vi "parseSpectralData.vi"(8 "error in (no error)":errorcluster, 11 "results-JSON string":string) -> (0 "error out":errorcluster, 2 "meta data":T1[][](array[typedef]), 3 "xyData":dbl[][][][](array[numeric]))   [LabVIEW 2023, in "CCD.lvclass"]
uses:
  CCD.lvclass
  CCDSpectralData.ctl
  81c9510d-da94-45eb-b341-4ac2c5dcdc17.vi
  <vilib>/JDP Science/JSONtext/Next JSON Value.vi
  <vilib>/JDP Science/JSONtext/String Subset.vi
  <vilib>/JDP Science/JSONtext/Parsing/Advance past next JSON Value (inlined COPY).vi
  <vilib>/JDP Science/JSONtext/Parsing/Advance past whitespace.vi
  <vilib>/JDP Science/JSONtext/Parsing/Advance past String.vi
  <vilib>/JDP Science/JSONtext/Parsing/Advance past Number.vi
  <vilib>/JDP Science/JSONtext/Parsing/Advance past Line Ending.vi
  <vilib>/JDP Science/JSONtext/Parsing/Parse Full Path or Item Name.vi
  <vilib>/JDP Science/JSONtext/Parsing/Advance past Array.vi
  <vilib>/JDP Science/JSONtext/Parsing/Advance past Object.vi
  <vilib>/JDP Science/JSONtext/support/Error Cluster From Code.vi
  <vilib>/JDP Science/JSONtext/Offset/Find Item Locations by Path.vi
  <vilib>/JDP Science/JSONtext/JSON text to Variant.vi
  <vilib>/JDP Science/JSONtext/LVClass Serializer/JSONtext LVClass Serializer.lvclass
  CCD.lvclass/CCD.ctl
  <vilib>/JDP Science/JSONtext/JSONtext.lvlib
panel:
  # "acquisition"
  # "ROI"
  # "x-pixel (wavelength)"
  # "unused"
  # "Connector Pane"
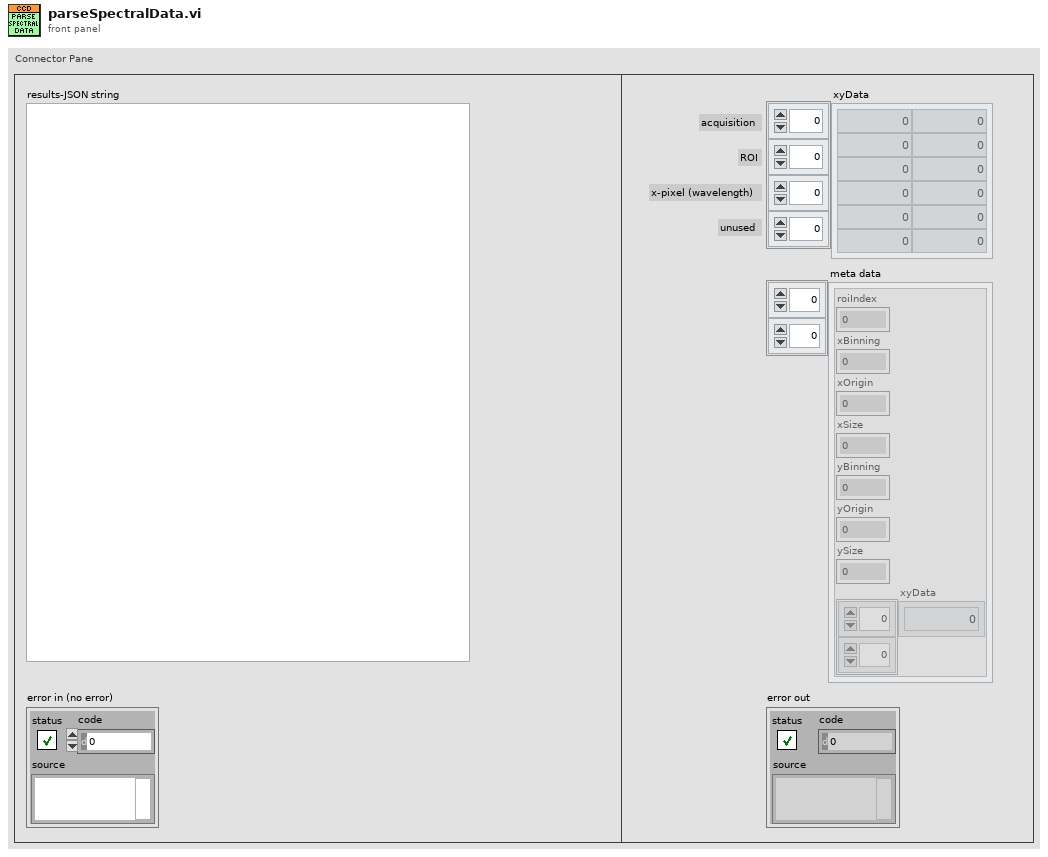
[diagram p1: front panel]
types:
  T1 = typedef "CCD.lvclass/CCDSpectralData.ctl" = cluster{"roiIndex":i32, "xBinning":i32, "xOrigin":i32, "xSize":i32, "yBinning":i32, "yOrigin":i32, "ySize":i32, "xyData":dbl[][]}
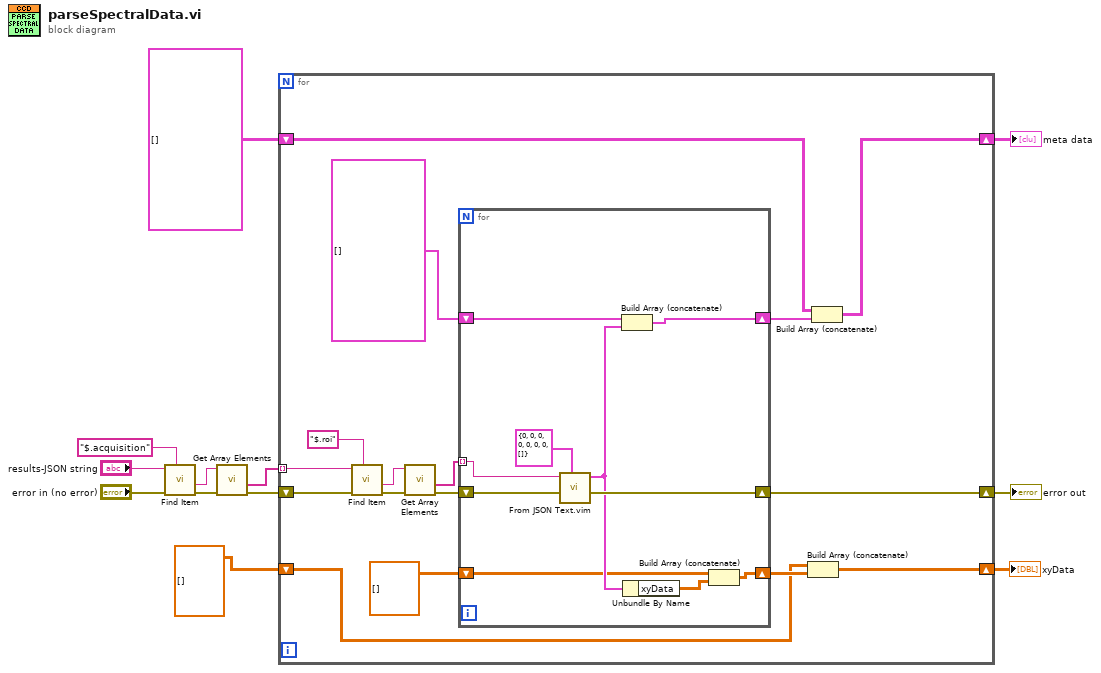
[diagram p0: block diagram]
diagram:
  n1 = call <vilib>:"Find Item.vi"("$Path or Item Name"="$.acquisition", "error in (no error)"="error in (no error)", "JSON"="results-JSON string") -> ("error out"=w9:errorcluster, "<JSON>"=w8:string)  [unwired: 5 in, 2 out]
  n2 = call <vilib>:"Get Array Elements.vi"("error in (no error)"=w9, "JSON"=w8) -> ("error out"=w12:errorcluster, "<JSON>"=w11:string[])  [unwired: 7 in, 1 out]
  n3 = for {
    tunnel: w11 -> [w22] mode=indexing
    shift-right: [w23] -> w7
    shift-left: w12 -> [w25]
    shift-right: [w17] -> w3
    shift-left: T1[][] [] -> [w18]
    shift-right: [w14] -> w1
    shift-left: dbl[][][][] [] -> [w13]
    n4 = call <vilib>:"Find Item.vi"("$Path or Item Name"="$.roi", "error in (no error)"=w25, "JSON"=w22) -> ("error out"=w27:errorcluster, "<JSON>"=w26:string)  [unwired: 5 in, 2 out]
    n5 = call <vilib>:"Get Array Elements.vi"("error in (no error)"=w27, "JSON"=w26) -> ("error out"=w24:errorcluster, "<JSON>"=w21:string[])  [unwired: 7 in, 1 out]
    n6 = for {
      shift-right: [w34] -> w23
      shift-left: w24 -> [w35]
      tunnel: w21 -> [w33] mode=indexing
      shift-right: [w37] -> w19
      shift-left: T1[] [] ("Array") -> [w36]
      shift-right: [w29] -> w15
      shift-left: dbl[][][] [] -> [w30]
      n7 = call "From JSON Text.vim"("Data Type and Default Value"=T1 {"roiIndex"=0, "xBinning"=0, "xOrigin"=0, "xSize"=0, "yBinning"=0, "yOrigin"=0, "ySize"=0, "xyData"=[]} ("Gain"), "error in (no error)"=w35, "JSON"=w33) -> ("error out"=w34:errorcluster, "Data out"=w32:T1)  [unwired: 7 in]
      n8 = Build Array (concatenate)(w36, w32) -> (w37:T1[])
      n9 = Unbundle By Name(w32) -> ("xyData"=w31:dbl[][])
      n10 = Build Array (concatenate)(w30, w31) -> (w29:dbl[][][])
    }
    n11 = Build Array (concatenate)(w13, w15) -> (w14:dbl[][][][])
    n12 = Build Array (concatenate)(w18, w19) -> (w17:T1[][])
  }
  "error out" <- w7
  "xyData" <- w1
  "meta data" <- w3
